vi "opencvFindPeak.vi"(2 "blur":dbl=1.0, 3 "Image (2D)":u16[][](array[numeric])) -> (0 "maxLocY":i32, 1 "maxLocX":i32)   [LabVIEW 2017]
uses:
  dll/wormUtilities/x64/Release/wormUtilities.dll
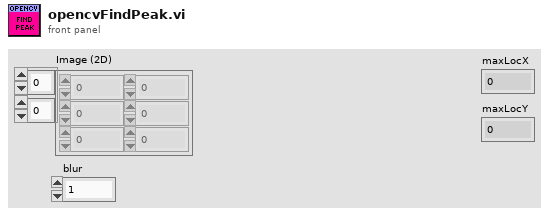
[diagram p1: front panel]
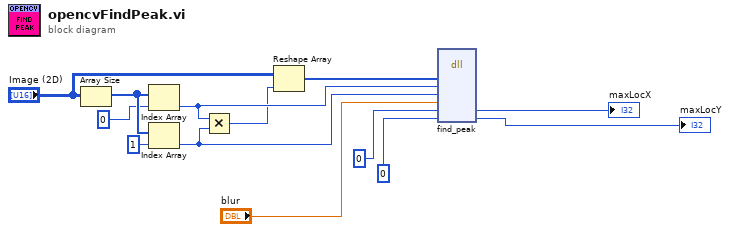
[diagram p0: block diagram]
diagram:
  n1 = Array Size(array="Image (2D)") -> (size(s)=w11:i32[])
  n2 = Index Array(array=w11, index=0) -> (element=w3:i32)
  n3 = Index Array(array=w11, index=1) -> (element=w2:i32)
  n4 = Multiply(x=w3, y=w2) -> (x*y=w1:i32)
  n5 = Reshape Array("Image (2D)", w1) -> (w8:u16[])
  n6 = dll-call lib="C:/Users/francesco/dev/pump-probe/dll/wormUtilities/x64/Release/wormUtilities.dll" fn="find_peak"("ImgIn"=w8, "sizex"=w3, "sizey"=w2, "blur"="blur", "maxLocX"=0, "maxLocY"=0) -> ("maxLocX"=→"maxLocX":i32, "maxLocY"=→"maxLocY":i32)  [unwired: 8 in, 2 out]
